vi "AI color scada short.vi"(8 "error in":errorcluster, 9 "change":bool, 10 "AIState":T1[](array[typedef]), 11 "AI_refs":refnum<vi>[](array[refnum])) -> (0 "error":errorcluster)   [LabVIEW 2019, in "Inputs.lvlib"]
uses:
  Inputs.lvlib
  Ctl/Parameter State short.ctl
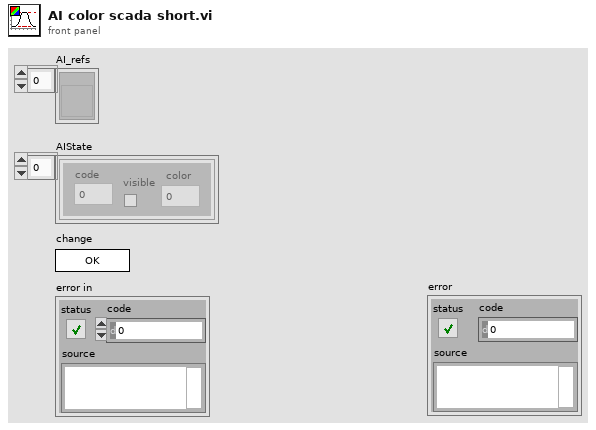
[diagram p1: front panel]
types:
  T1 = typedef "Inputs.lvlib/Parameter State short.ctl" = cluster{"code":i32, "visible":bool, "color":u32}
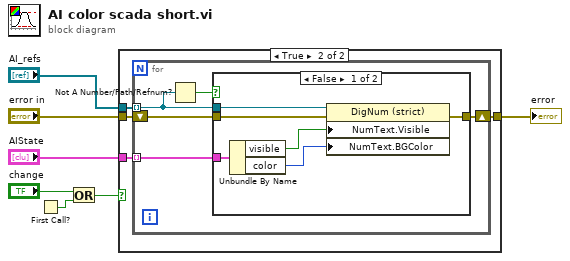
[diagram p0: block diagram]
diagram:
  n1 = First Call?() -> (First Call?: T/F=w1:bool)
  n2 = Or(x="change", y=w1) -> (x .or. y?=w2:bool)
  n3 = case shown="True" w2 {
    tunnel: [w8 w12] -> w4
    tunnel: "error in" -> [w8 w11]
    tunnel: "AI_refs" -> [_ w10]
    tunnel: "AIState" -> [_ w9]
    frame False {
    }
    frame True {
      n4 = for {
        tunnel: w10 -> [w14] mode=indexing
        tunnel: w9 -> [w17] mode=indexing
        shift-right: [w15] -> w12
        shift-left: w11 -> [w16]
        n5 = Not A Number/Path/Refnum?(number/path/refnum=w14) -> (NaN/Path/Refnum?=w13:bool)
        n6 = case shown="False" w13 {
          tunnel: w17 -> [w23 _]
          tunnel: w16 -> [w22 w24]
          tunnel: [w21 w24] -> w15
          tunnel: w14 -> [w20 _]
          frame False {
            n7 = Unbundle By Name(w23) -> ("visible"=w19:bool, "color"=w18:u32)
            n8 = property on="Property Node" class="DigNum (strict)"(reference=w20, error in=w22, "NumText.Visible"=w19, "NumText.BGColor"=w18) -> (error out=w21:errorcluster)  [unwired: 1 out]
          }
          frame True {
          }
        }
      }
    }
  }
  "error" <- w4
